vi "DllFxpRectToPolarTemp.vi"(6 "ready for output":bool, 9 "input valid":bool, 10 "x":fxp<+/-,64,32>, 11 "y":fxp<+/-,64,32>) -> (1 "output valid":bool, 2 "phase":fxp<+,1,1>, 3 "magnitude":fxp<+,1,1>, 4 "ready for input":bool)   [LabVIEW 2017]
uses:
  <vilib>/rvi/FXPMathLib/FxpRectToPolar/subVIs/nifxpmath_RectToPolar_SimConfig.ctl
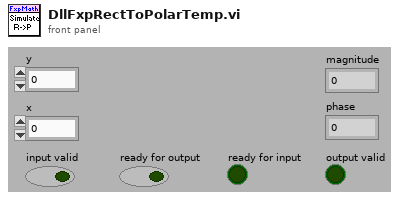
[diagram p1: front panel]
types:
  T1 = typedef "nifxpmath_RectToPolar_SimConfig.ctl" = cluster{"kXSigned":bool, "kXWl":u32, "kXIwl":i32, "kYSigned":bool, "kYWl":u32, "kYIwl":i32, "kPhaseLen":u16, "kPhaseIwl":i16, "kMagnitudeLen":u16, "internal xy wl":u16, "internal xy iwl":i16, "kCoarseRotation":bool, "kPrecision":u16, "kIteration":u16, "kQuaMode":u16, "kInsideSCTL":bool, "kCycleLimit":u16, "kStrictLimit":bool, "InputRegister":bool, "OutputRegister":bool, "kGainCompst":bool, "kExtraCycle":bool}
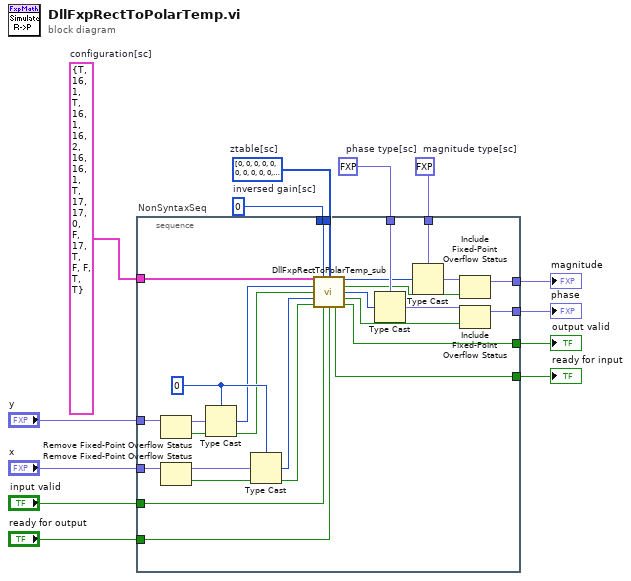
[diagram p0: block diagram]
diagram:
  w1 = T1 {"kXSigned"=TRUE, "kXWl"=16, "kXIwl"=1, "kYSigned"=TRUE, "kYWl"=16, "kYIwl"=1, "kPhaseLen"=16, "kPhaseIwl"=2, "kMagnitudeLen"=16, "internal xy wl"=16, "internal xy iwl"=1, "kCoarseRotation"=TRUE, "kPrecision"=17, "kIteration"=17, "kQuaMode"=0, "kInsideSCTL"=FALSE, "kCycleLimit"=17, "kStrictLimit"=TRUE, "InputRegister"=FALSE, "OutputRegister"=FALSE, "kGainCompst"=TRUE, "kExtraCycle"=TRUE}  # configuration[sc]
  w7 = fxp<+,1,1> 0.0  # phase type[sc]
  w10 = fxp<+,1,1> 0.0  # magnitude type[sc]
  w6 = u64 0  # inversed gain[sc]
  w5 = u64[] [0, 0, 0, 0, 0, 0, 0, 0, 0, 0, 0, 0, 0, 0, 0, 0]  # ztable[sc]
  n1 = stacked-sequence "NonSyntaxSeq" {
    tunnel: "input valid" -> [w26]
    tunnel: "y" -> [w34]
    tunnel: "x" -> [w32]
    tunnel: w10 -> [w39]
    tunnel: [w17] -> w9
    tunnel: [w16] -> w8
    tunnel: w7 -> [w37]
    tunnel: w6 -> [w36]
    tunnel: w5 -> [w35]
    tunnel: "ready for output" -> [w25]
    tunnel: [w24] -> w2
    tunnel: [w15] -> w3
    tunnel: w1 -> [w14]
    frame #0 {
      w38 = u64 0
      n2 = Remove Fixed-Point Overflow Status(3:w34) -> (0:w29:bool, 1:w33:fxp<+/-,64,32>)
      n3 = Remove Fixed-Point Overflow Status(3:w32) -> (0:w27:bool, 1:w31:fxp<+/-,64,32>)
      n4 = Type Cast(type=w38, x=w33) -> (*(type *) &x=w30:u64)
      n5 = Type Cast(type=w38, x=w31) -> (*(type *) &x=w28:u64)
      n6 = call <vilib>:"DllFxpRectToPolarTemp_sub.vi"("configuration[sc]"=w14, "inversed gain"=w36, "ztable"=w35, "y"=w30, "y ovfl status"=w29, "x"=w28, "x ovfl status"=w27, "input valid"=w26, "ready for output"=w25) -> ("magnitude"=w23:u64, "magnitude ovfl status"=w20:bool, "phase"=w22:u64, "phase ovfl status"=w18:bool, "ready for input"=w24:bool, "output valid"=w15:bool)  [unwired: 1 out]
      n7 = Type Cast(type=w37, x=w22) -> (*(type *) &x=w19:fxp<+,1,1>)
      n8 = Type Cast(type=w39, x=w23) -> (*(type *) &x=w21:fxp<+,1,1>)
      n9 = Include Fixed-Point Overflow Status(2:w20, 3:w21) -> (1:w17:fxp<+,1,1>)
      n10 = Include Fixed-Point Overflow Status(2:w18, 3:w19) -> (1:w16:fxp<+,1,1>)
    }
  }
  "output valid" <- w3
  "ready for input" <- w2
  "magnitude" <- w9
  "phase" <- w8
